vi "get data interface information.vi"(11 "System Diagnostics runtime in":refnum<class "System Diagnostics runtime.lvclass">) -> (2 "data type defs":T1, 3 "System Diagnostics runtime out":refnum<class "System Diagnostics runtime.lvclass">)   [LabVIEW 2013, in "System Diagnostics runtime.lvclass"]
uses:
  System Diagnostics runtime.lvclass
  <vilib>/NI/Tag Bus Data Framework/fixed module parent/module/execution/data cluster type definition.ctl
  output user data.ctl
  parameter user data.ctl
  result user data.ctl
  input user data.ctl
  <vilib>/NI/Tag Bus Data Framework/fixed module parent/module/execution/fixed channel runtime.lvclass
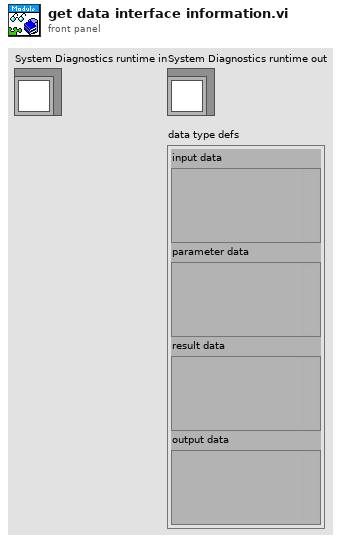
[diagram p1: front panel]
types:
  T1 = typedef "fixed channel runtime.lvclass/data cluster type definition.ctl" = cluster{"input data":variant, "parameter data":variant, "result data":variant, "output data":variant}
  T2 = typedef "System Diagnostics runtime.lvclass/input user data.ctl" = cluster{"CPU load average":dbl, "timed structures load":dbl, "free memory":dbl, "contiguous memory":dbl}
  T3 = typedef "System Diagnostics runtime.lvclass/result user data.ctl" = cluster{"fmwk_placeholder":i32}
  T4 = typedef "System Diagnostics runtime.lvclass/parameter user data.ctl" = cluster{"fmwk_placeholder":i32}
  T5 = typedef "System Diagnostics runtime.lvclass/output user data.ctl" = cluster{"fmwk_placeholder":i32}
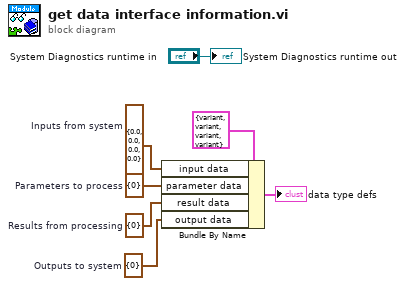
[diagram p0: block diagram]
diagram:
  w1 = T2 {"CPU load average"=0.0, "timed structures load"=0.0, "free memory"=0.0, "contiguous memory"=0.0}  # Inputs from system
  w3 = T3 {"fmwk_placeholder"=0}  # Results from processing
  w2 = T4 {"fmwk_placeholder"=0}  # Parameters to process
  w4 = T5 {"fmwk_placeholder"=0}  # Outputs to system
  n1 = Bundle By Name(cluster=T1 {"input data"=variant, "parameter data"=variant, "result data"=variant, "output data"=variant} ("data type defs"), "input data"=w1, "parameter data"=w2, "result data"=w3, "output data"=w4) -> (→"data type defs":T1)
  "System Diagnostics runtime out" <- "System Diagnostics runtime in"
